vi "secondaire.vi"() -> ()   [LabVIEW 2018]
uses:
  Global vars.vi
panel:
  in  "stop":bool
  in  "Phase 4":dbl
  in  "Phase 3":dbl
  in  "Phase 2":dbl
  in  "Phase 1":dbl
  # "Durée des phases en secondes"
  # "Phase 1"
  # "Phase 2"
  # "Phase 3"
  # "Phase 4"
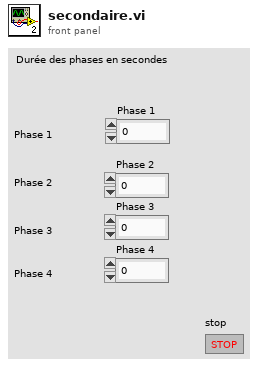
[diagram p1: front panel]
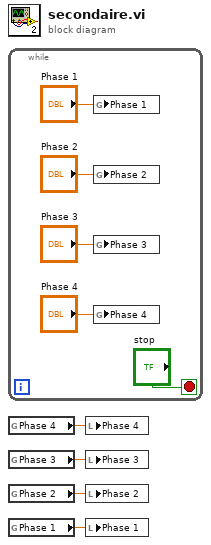
[diagram p0: block diagram]
diagram:
  n1 = while {
    stop <- "stop" stop-if-true
    n2 = global write "Global vars.vi" "Phase 1"("Phase 1") -> ()
    n3 = global write "Global vars.vi" "Phase 2"("Phase 2") -> ()
    n4 = global write "Global vars.vi" "Phase 3"("Phase 3") -> ()
    n5 = global write "Global vars.vi" "Phase 4"("Phase 4") -> ()
  }
  n6 = global read "Global vars.vi" "Phase 4"() -> (w4:dbl)
  n7 = global read "Global vars.vi" "Phase 3"() -> (w3:dbl)
  n8 = global read "Global vars.vi" "Phase 2"() -> (w2:dbl)
  n9 = global read "Global vars.vi" "Phase 1"() -> (w1:dbl)
  n10 = local write "Phase 4"(w4) -> ()
  n11 = local write "Phase 3"(w3) -> ()
  n12 = local write "Phase 2"(w2) -> ()
  n13 = local write "Phase 1"(w1) -> ()
